vi "Initiate.vi"(8 "error in (no error)":errorcluster {"code" format="%.0x"}, 11 "VISA resource name":refnum<visa-resource-name>) -> (0 "error out":errorcluster {"code" format="%.0x"}, 3 "VISA resource name out":refnum<visa-resource-name>)   [LabVIEW 2016, in "Agilent N6700 Series.lvlib"]
doc: "This VI initiates output changes that you previously specified.\n\nIf the power supply is not currently waiting for a trigger, the power supply waits for the trigger you specify with the agn6700 Configure Trigger Source.vi after you call this VI. After the power supply detects the trigger, it updates its voltage level and current limit to the values you specify with the agn6700 Configure Triggered Voltage Lev.vi and agn6700 Configure Triggered Current Lim.vi VIs.\n\nIf the power supply is already waiting for a trigger, this VI does nothing and returns VI_SUCCESS.\n\n\n<b>Note:</b>\n\nDoes not abort individual channels.\n\nThis VI can generate an error with double modules."
uses:
  <instrlib>/Agilent N6700 Series/Agilent N6700 Series.lvlib
panel:
  # "Note:\nThis VI has been obsoleted from the driver and is included for compatibility with existing applications.  New applications should use the Initiate Output Trigger VI"
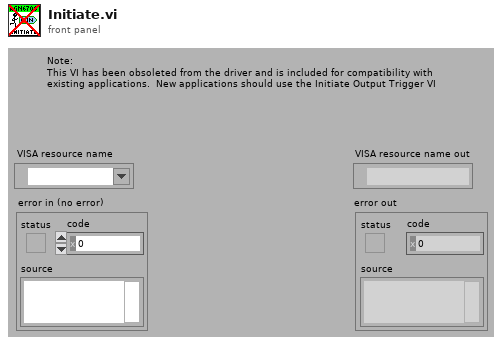
[diagram p1: front panel]
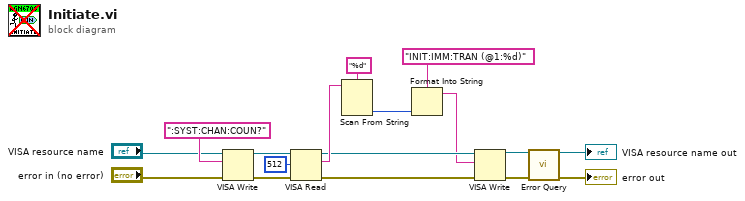
[diagram p0: block diagram]
diagram:
  n1 = VISA Write(VISA resource name="VISA resource name", write buffer=":SYST:CHAN:COUN?", error in (no error)="error in (no error)") -> (VISA resource name out=w11:refnum<visa-resource-name>, error out=w12:errorcluster)  [unwired: 1 out]
  n2 = VISA Read(VISA resource name=w11, byte count=u32 512, error in (no error)=w12) -> (VISA resource name out=w9:refnum<visa-resource-name>, read buffer=w15:string, error out=w10:errorcluster)  [unwired: 1 out]
  n3 = Scan From String(format string="%d", input string=w15) -> (output 1=w7:i32)  [unwired: 3 in, 3 out]
  n4 = Format Into String(format string="INIT:IMM:TRAN (@1:%d)", w7) -> (resulting string=w5:string)  [unwired: 2 in, 1 out]
  n5 = VISA Write(VISA resource name=w9, write buffer=w5, error in (no error)=w10) -> (VISA resource name out=w2:refnum<visa-resource-name>, error out=w1:errorcluster)  [unwired: 1 out]
  n6 = call <instrlib>:"Error Query.vi"("VISA resource name"=w2, "error in (no error)"=w1) -> ("VISA resource name out"=→"VISA resource name out":refnum<visa-resource-name>, "error out"=→"error out":errorcluster)  [unwired: 10 in, 2 out]
